vi "lab #5 (while loop).vi"() -> ()   [LabVIEW 2016]
panel:
  out "Numeric":i32
  in  "y":bool
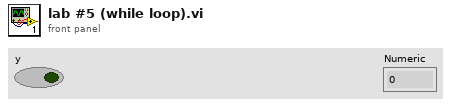
[diagram p1: front panel]
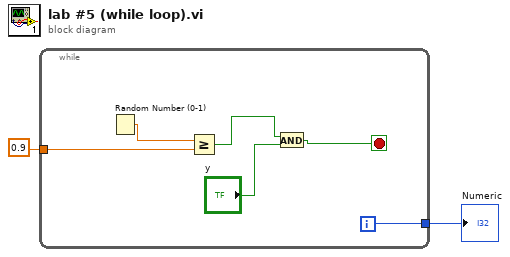
[diagram p0: block diagram]
diagram:
  n1 = while {
    tunnel: 0.9 ("x") -> [w7]
    tunnel: [w4] -> w1
    i -> [w4]
    stop <- w5 stop-if-true
    n2 = Random Number (0-1)() -> (number: 0 to 1=w8:dbl)
    n3 = Greater Or Equal?(x=w8, y=w7) -> (x >= y?=w6:bool)
    n4 = And(x=w6, y="y") -> (x .and. y?=w5:bool)
  }
  "Numeric" <- w1
